vi "8-Tap 8-bit Camera with Serial Server(FPGA).vi"() -> ()   [LabVIEW 2013]
doc: "This is the FPGA VI for the 10-Tap 8-Bit Camera with DRAM example. This example demonstrates how to acquire images from a 10-tap, 8-bit, extended configuration, Camera Link camera and transfer the images to the host. This example supports area scan and line scan cameras for both continuous and finite acquisitions.\n\nThis example also demonstrates the use of DRAM as a frame buffer for very high speed acquisitions. Data packing and flow-control are also employed to maximize use of the available DRAM and FIFOs in terms of both memory space and performance.\n\nAdditionally, the example demonstrates the serial server, which allows third-party camera configuration utilities to communicate with the camera using the Camera Link serial interface while this VI is running."
uses:
  Common/CL Signal Mapping.ctl
  Common/CL Configuration.ctl
  FPGA/Sector/Accumulate/Sector Parameter Cluster.ctl
  <vilib>/Platform/TimedLoop/XDataNode/timing_clust.ctl
  <vilib>/Platform/TimedLoop/XDataNode/nitl_modes.ctl
  <vilib>/Platform/TimedLoop/XDataNode/wakeup.ctl
  <vilib>/rvi/Emulation/niFpgaSctlEmulationGetInTimedLoop.vi
  <vilib>/rvi/Emulation/niFpgaEmulationReportErrorSimple.vi
  <vilib>/rvi/eio/common/nirviEmuTemplateMethod_errors.vi
  <vilib>/rvi/Emulation/niFpgaGetClockAttributes.vi
  <vilib>/rvi/Emulation/niFpgaCriticalErrorInLSC.vi
  FPGA/Globals/Sector Parameter Global.vi
  Common/CL Data to Pixels/8 Tap 8-Bit.vi
  <vilib>/rvi/FIFO/Fifo_Resource/nirvififoEmulationWriteFpgaImpl.vi
  <vilib>/rvi/DataTransferAndStorage/Container/Common/niFpgaContainerGetUniqueNameForEmu.vi
  <vilib>/rvi/interface/RandomDataEmulation/nirviRandomDataFPGAFIFO.vi
  <vilib>/rvi/interface/RandomDataEmulation/niFpgaRandomDataHandleErrors.vi
  <vilib>/rvi/FIFO/Fifo_Resource/nirvififoEmulationGetNumberOfElementsToReadFpgaImpl.vi
  <vilib>/rvi/FIFO/Fifo_Resource/nirvififoEmulationGetNumberOfElementsToWriteFpgaImpl.vi
  <vilib>/rvi/FIFO/Fifo_Resource/nirvififoEmulationReadFpgaImpl.vi
  <vilib>/rvi/Emulation/niFpgaProcessEmulError.vi
  FPGA/Globals/Pixel Location Global.vi
  FPGA/Globals/Accumulated Sector Intensity.vi
  <vilib>/Platform/TimedLoop/XDataNode/XDataNode.xnode
  <vilib>/eio/EIONode/EIONode.xnode
  <vilib>/rvi/DataTransferAndStorage/Container/XNode/niFpgaContainer.xnode
  <vilib>/rvi/FIFO/Fifo_Resource/nirvififoEmulationWrite.vi
  <vilib>/rvi/interface/RandomDataEmulation/nirviRandomDataFpgaReadWriteTemplate.vi
  <vilib>/rvi/FIFO/Fifo_Resource/nirvififoEmulationGetNumberOfElementsToRead.vi
  <vilib>/rvi/FIFO/Fifo_Resource/nirvififoEmulationGetNumberOfElementsToWrite.vi
  <vilib>/rvi/FIFO/Fifo_Resource/nirvififoEmulationRead.vi
  <vilib>/Platform/TimedLoop/XDataNode/XDNodeRunTimeDep.lvlib
panel:
  out "Analysis Ticks":u32
  out "Right Sector Edge":u8
  out "Left Sector Edge":u8
  in  "# of Frames to Average":u8
  in  "Sector Parameters Left":T1={"Start Angle"=0.65740966796875, "End Angle"=0.99468994140625, "Inner Radius"=309, "Outter Radius"=405, "Hinge X"=464, "Hinge Y"=534, "NumWingSectors"=8}
  in  "Sector Parameters Right":T1={"Start Angle"=0.0, "End Angle"=0.4708251953125, "Inner Radius"=309, "Outter Radius"=405, "Hinge X"=685, "Hinge Y"=527, "NumWingSectors"=8}
  in  "Sector Threshold":u8
  in  "[Average BG Intensity]":u8[](array[numeric])=[0, 0, 0, 0, 0, 0, 0, 0, 0, 0, 0, 0, 0, 0, 0, 0, 0, 0, 0, 0, 0, 0, 0, 0, 0, 0, 0, 0, 0, 0, 0, 0]
  in  "X Resolution":u16=1000
  in  "Y Resolution":u16=1000
  in  "Left Start Angle Duty Cycle":fxp<+,8,0>
  in  "Left End Angle Duty Cycle":fxp<+,8,0>
  in  "Right Start Angle Duty Cycle":fxp<+,8,0>
  in  "Right End Angle Duty Cycle":fxp<+,8,0>
  out "Number of Elements to Write Host DMA":u32
  out "Number of Elements to Read Cam Data":u32
  in  "CL Config.Configuration":T2=enum."Full"
  in  "CL Config.Signal Mapping":T3
  in  "CL Config.Line Scan":bool
  in  "CL Config.DVAL Active High":bool=TRUE
  in  "CL Config.LVAL Active High":bool=TRUE
  in  "CL Config.FVAL Active High":bool=TRUE
  in  "CL Config.Spare Active High":bool=TRUE
  in  "Acq Control.Line Scan Height":u32
  in  "Acq Control.Frames To Acq":u32
  in  "Acq Control.Acquire":bool
  in  "Acq Control.Cancel Acq":bool
  in  "Acq Control.Ignore DVAL":bool
  in  "Acq Control.Initialize":bool
  out "Acq Status.Acq In Progress":bool
  out "Acq Status.Clocks Per Line":u32
  out "Acq Status.Frames Acq'd":u32
  out "Acq Status.Lines Per Frame":u32
  out "Acq Status.DMA Write Timeout":bool
  out "Acq Status.Initialized":bool
  in  "UART.Baud Rate":u8
  in  "UART.Transmit":bool
  in  "UART.Tx Data":u8[](array[numeric])=[0, 0, 0, 0, 0, 0, 0, 0, 0, 0] format="%02x"
  in  "UART.Set Baud Rate":bool
  in  "UART.Byte Mode":bool=TRUE
  out "UART.Rx Ready":bool
  out "UART.Break Indicator":bool
  out "UART.Framing Error":bool
  out "UART.Overrun Error":bool
  out "UART.Tx Ready":bool
  out "UART.Rx Data":u8 format="%02x"
  in  "UART.Receive":bool
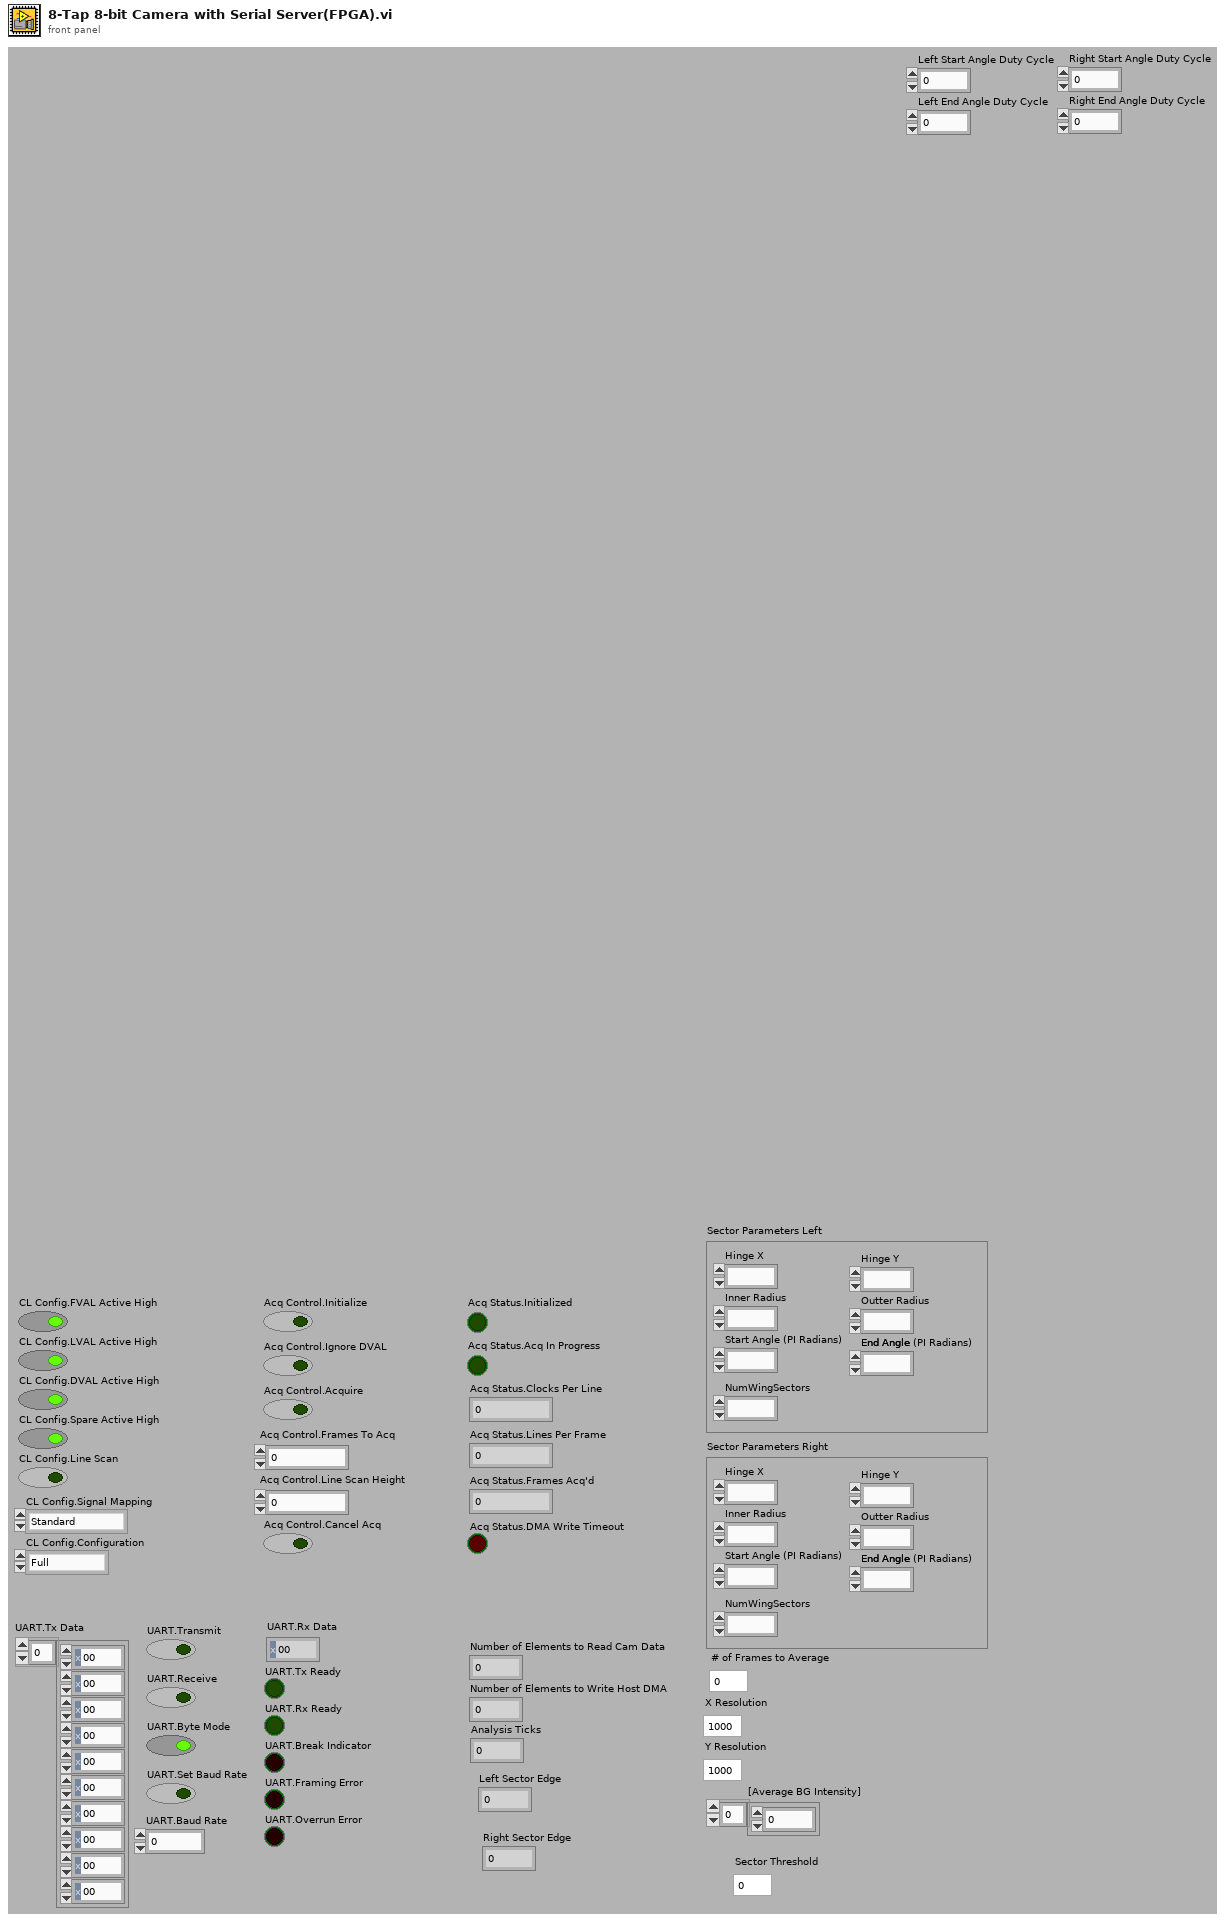
[diagram p1: front panel]
types:
  T1 = typedef "Sector Parameter Cluster.ctl" = cluster{"Start Angle":fxp<+/-,17,2>, "End Angle":fxp<+,17,3>, "Inner Radius":u16, "Outter Radius":u16, "Hinge X":u16, "Hinge Y":u16, "NumWingSectors":u8}
  T2 = typedef "CL Configuration.ctl" = enum8{"Base", "Medium", "Full"}
  T3 = typedef "CL Signal Mapping.ctl" = enum8{"Standard", "Basler 10-tap", "Vosskühler 10-tap"}
  T4 = typedef "XDNodeRunTimeDep.lvlib/timing_clust.ctl" = cluster{"Expected End [f-1]":u64, "Actual End [f-1]":u64, "Finished Late? [f-1]":bool, "Expected End [i-1]":u64, "Actual End [i-1]":u64, "Finished Late? [i-1]":bool, "Expected Start [i]":u64, "Actual Start [i]":u64, "Expected Start [f]":u64, "Actual Start [f]":u64, "Source Name":string, "Structure Name":string, "Period":i64, "Deadline":i64, "Offset":i64, "Start":i64, "Priority":i32, "Timeout":i32, "Mode":T5, "Wakeup Reason":T6, "Error":errorcluster, "Source Type":string, "Secondary Source Type":string, "Global End Time":u64, "Global Start Time":u64, "Frame Duration":u64, "Iteration Duration":u64, "Assigned CPU":i32, "I/O Scan Engine Mode":u32}
  T5 = typedef "XDNodeRunTimeDep.lvlib/nitl_modes.ctl" = enum32{"No Change", "Process missed periods, maintain original phase", "Discard missed periods, maintain original phase", "Process missed periods, ignore original phase", "Discard missed periods, ignore original phase"}
  T6 = typedef "XDNodeRunTimeDep.lvlib/wakeup.ctl" = enum32{"Normal", "Aborted", "Asynchronous wakeup", "Timing source error", "Timed loop error", "Timeout"}
  T7 = cluster{"Enables Valid":bool, "Frame Valid":bool, "Line Valid":bool, "Data Valid":bool}
  T8 = cluster{"Pixel 0":u8, "Pixel 1":u8, "Pixel 2":u8, "Pixel 3":u8, "Pixel 4":u8, "Pixel 5":u8, "Pixel 6":u8, "Pixel 7":u8}
  T9 = cluster{"Tx Data":u8[], "Transmit":bool, "Receive":bool, "Byte Mode":bool, "Set Baud Rate":bool, "Baud Rate":u8}
  T10 = cluster{"Rx Data":u8, "Turn Off Transmit":bool, "Turn Off Receive":bool, "Turn Off Set Baud Rate":bool, "Tx Ready":bool, "Rx Ready":bool, "Break Indicator":bool, "Framing Error":bool, "Overrun Error":bool}
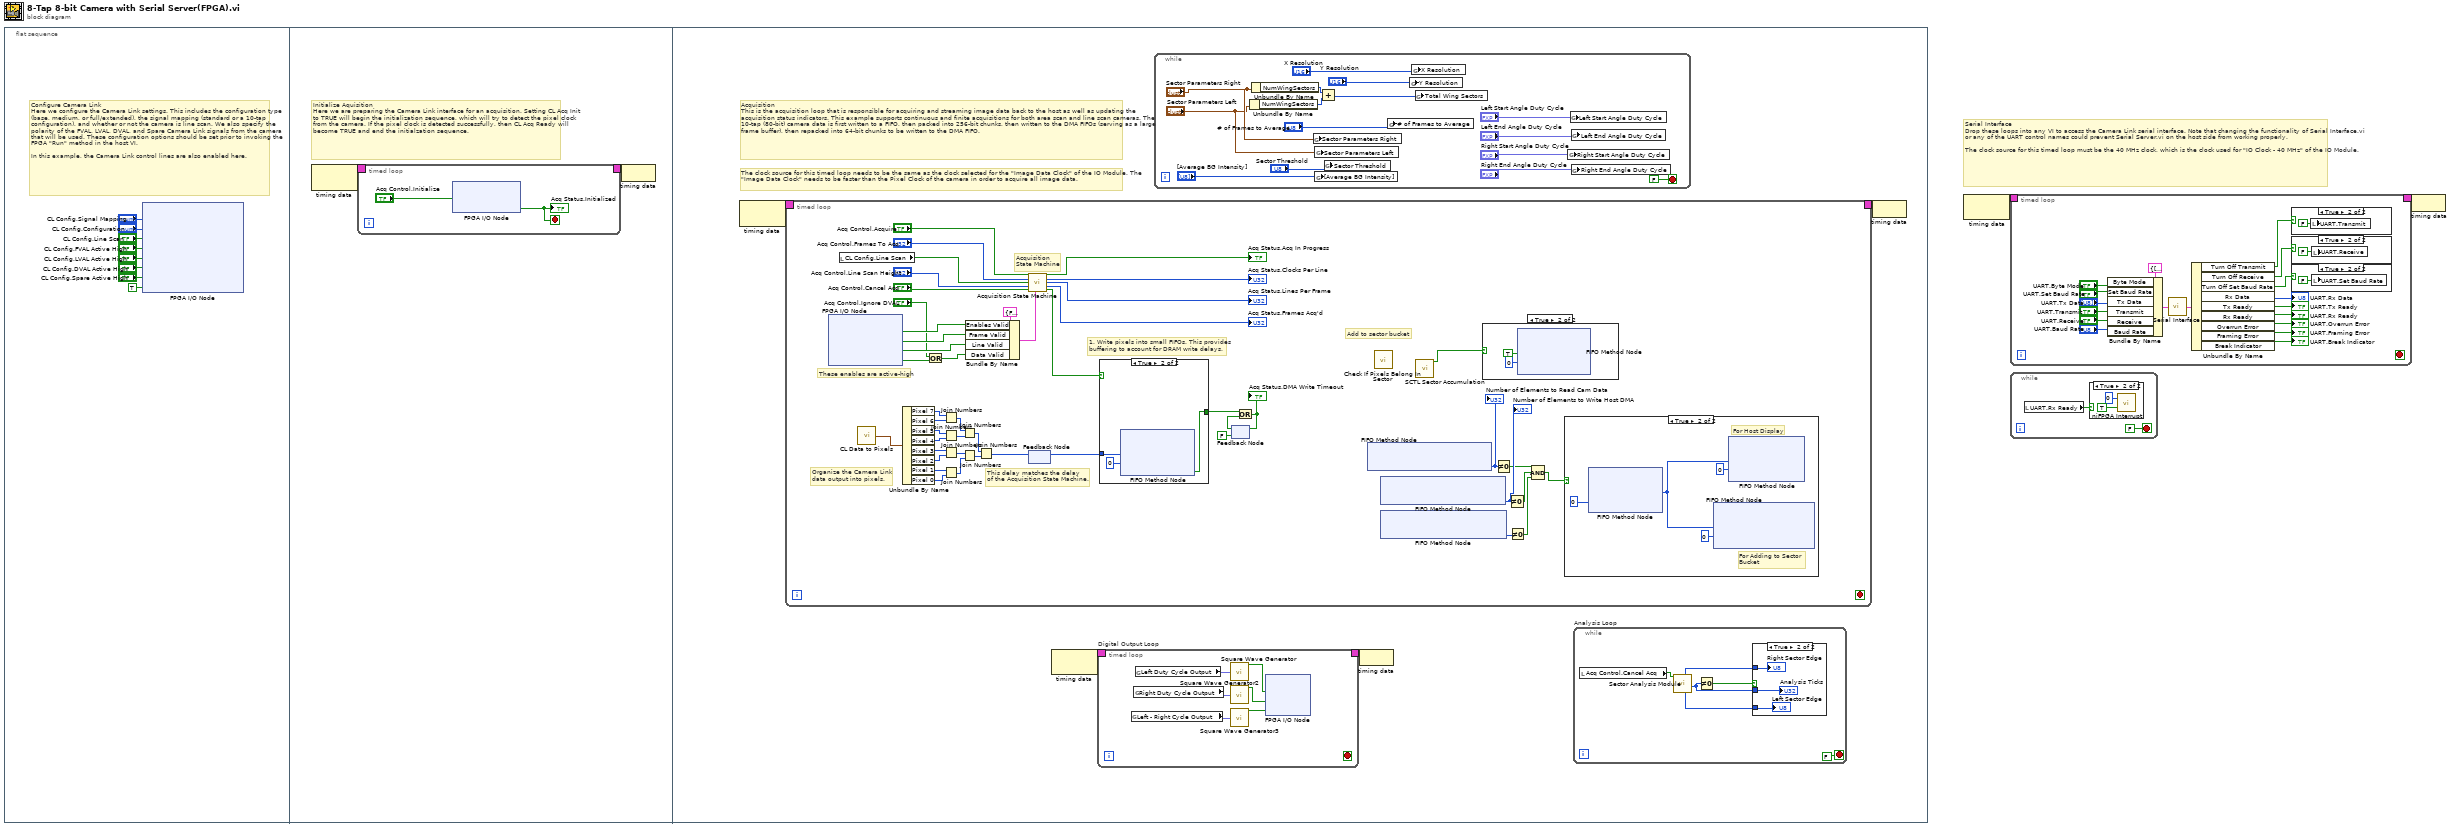
[diagram p0: block diagram]
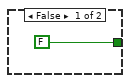
[diagram p9: hidden frame]
diagram:
  # "Serial Interface\nDrop these loops into any VI to access the Camera Link serial interface. Note that changing the functionality of Serial Interface.vi or any of the UART control names could prevent Serial Server.vi on the host side from working properly.\n\nThe clock source for this timed loop must be the 40 MHz clock, which is the clock used for \"IO Clock - 40 MHz\" of the IO Module."
  n1 = flat-sequence {
    frame #0 {
      # "Configure Camera Link\nHere we configure the Camera Link settings. This includes the configuration type (base, medium, or full/extended), the signal mapping (standard or a 10-tap configuration), and whether or not the camera is line scan. We also specify the polarity of the FVAL, LVAL, DVAL, and Spare Camera Link signals from the camera that will be used. These configuration options should be set prior to invoking the FPGA \"Run\" method in the host VI.\n\nIn this example, the Camera Link control lines are also enabled here."
      n2 = xnode "FPGA I/O Node"("CL Set Signal Mapping"="CL Config.Signal Mapping", "CL Set Configuration"="CL Config.Configuration", "CL Set Line Scan"="CL Config.Line Scan", "CL Set FVAL Active High"="CL Config.FVAL Active High", "CL Set LVAL Active High"="CL Config.LVAL Active High", "CL Set DVAL Active High"="CL Config.DVAL Active High", "CL Set Spare Active High"="CL Config.Spare Active High", "CL Control Enable"=TRUE ("IO Module\\CL Control Enable")) -> ()  [unwired: 8 in, 8 out]
    }
    frame #1 {
      # "Initialize Aquisition\nHere we are preparing the Camera Link interface for an acquisition. Setting CL Acq Init to TRUE will begin the initialization sequence, which will try to detect the pixel clock from the camera. If the pixel clock is detected successfully, then CL Acq Ready will become TRUE and end the initialzation sequence."
      n3 = node-c288() -> (w12:T4)  [unwired: 1 out]
      n4 = timed-loop {
        timing: w12 -> [_]
        timing-out: [_] -> w11
        stop <- w13 stop-if-true
        n5 = xnode "FPGA I/O Node"("CL Acq Init"="Acq Control.Initialize") -> ("CL Acq Ready"=w13:bool)  [unwired: 2 in, 2 out]
        "Acq Status.Initialized" <- w13
      }
      n6 = node-c288(w11) -> ()
    }
    frame #2 {
      # "The clock source for this timed loop needs to be the same as the clock selected for the \"Image Data Clock\" of the IO Module. The \"Image Data Clock\" needs to be faster than the Pixel Clock of the camera in order to acquire all image data."
      # "Acquisition\nThis is the acquisition loop that is responsible for acquiring and streaming image data back to the host as well as updating the acquisition status indicators. This example supports continuous and finite acquisitions for both area scan and line scan cameras. The 10-tap (80-bit) camera data is first written to a FIFO, then packed into 256-bit chunks, then written to the DMA FIFOs (serving as a large frame buffer), then repacked into 64-bit chunks to be written to the DMA FIFO."
      n7 = node-c288() -> (w22:T4)  [unwired: 1 in]
      n8 = timed-loop {
        timing: w22 -> [_]
        timing-out: [_] -> w21
        stop <- _ stop-if-true
        # "Add to sector bucket"
        # "1. Write pixels into small FIFOs. This provides\nbuffering to account for DRAM write delays."
        # "Organize the Camera Link\ndata output into pixels."
        # "These enables are active-high"
        # "This delay matches the delay\nof the Acquisition State Machine."
        # "Acquisition\nState Machine"
        n9 = xnode "FPGA I/O Node"() -> ("CL Output Valid"=w89:bool, "CL Frame Valid"=w88:bool, "CL Line Valid"=w87:bool, "CL Data Valid"=w84:bool)  [unwired: 4 in, 4 out]
        n10 = local read "CL Config.Line Scan"() -> (w81:bool)
        n11 = call-poly "CL Data to Pixels.vi"() -> ("Pixels"=w103:T8)  [unwired: 1 in]
        n12 = Unbundle By Name(w103) -> ("Pixel 7"=w79:u8, "Pixel 6"=w78:u8, "Pixel 5"=w77:u8, "Pixel 4"=w76:u8, "Pixel 3"=w75:u8, "Pixel 2"=w74:u8, "Pixel 1"=w73:u8, "Pixel 0"=w72:u8)
        n13 = Or(x="Acq Control.Ignore DVAL", y=w84) -> (x .or. y?=w83:bool)
        n14 = Join Numbers(hi=w79, lo=w78) -> ((hi.lo)=w70:u16)
        n15 = Join Numbers(hi=w77, lo=w76) -> ((hi.lo)=w69:u16)
        n16 = Join Numbers(hi=w75, lo=w74) -> ((hi.lo)=w68:u16)
        n17 = Join Numbers(hi=w73, lo=w72) -> ((hi.lo)=w71:u16)
        n18 = Join Numbers(hi=w70, lo=w69) -> ((hi.lo)=w67:u32)
        n19 = Join Numbers(hi=w68, lo=w71) -> ((hi.lo)=w66:u32)
        n20 = Bundle By Name(cluster=T7 {"Enables Valid"=FALSE, "Frame Valid"=FALSE, "Line Valid"=FALSE, "Data Valid"=FALSE} ("Enables"), "Enables Valid"=w89, "Frame Valid"=w88, "Line Valid"=w87, "Data Valid"=w83) -> (w86:T7)
        n21 = Join Numbers(hi=w67, lo=w66) -> ((hi.lo)=w65:u64)
        n22 = call "Acquisition State Machine.vi"("Acquire"="Acq Control.Acquire", "Frames to Acquire"="Acq Control.Frames To Acq", "Line Scan"=w81, "Line Scan Height"="Acq Control.Line Scan Height", "Cancel Acq"="Acq Control.Cancel Acq", "Enables"=w86) -> ("Acq In Progress"=→"Acq Status.Acq In Progress":bool, "Num Clocks Per Line"=→"Acq Status.Clocks Per Line":u32, "Num Lines Per Frame"=→"Acq Status.Lines Per Frame":u32, "Num Frames Acq'd"=→"Acq Status.Frames Acq'd":u32, "Capture Cycle"=w101:bool)  [unwired: 4 in, 1 out]
        n23 = feedback-in #1(w65) -> ()
        n24 = feedback #1() -> (w102:u64)  [unwired: 1 in]
        n25 = case shown="True" w101 {
          tunnel: [FALSE ("Timed Out?") w112] -> w99
          tunnel: w102 -> [_ w113]
          frame False {
          }
          frame True {
            n26 = xnode ("FIFO Method Node")("Element"=w113, "Timeout"=0) -> ("Timed Out?"=w112:bool)  [unwired: 1 in, 1 out]
          }
        }
        n27 = feedback #2(FALSE) -> (w98:bool)
        n28 = Or(x=w99, y=w98) -> (x .or. y?=w97:bool)
        "Acq Status.DMA Write Timeout" <- w97
        n29 = feedback-in #2(w97) -> ()
        n30 = xnode ("FIFO Method Node")() -> ("Number of Elements to Read"=w63:u32)  [unwired: 1 in, 1 out]
        "Number of Elements to Read Cam Data" <- w63
        n31 = call "Check If Pixels Belong In Sector.vi"() -> ()  [unwired: 11 in, 1 out]
        n32 = xnode ("FIFO Method Node")() -> ("Number of Elements to Write"=w61:u32)  [unwired: 1 in, 1 out]
        "Number of Elements to Write Host DMA" <- w61
        n33 = xnode ("FIFO Method Node")() -> ("Number of Elements to Write"=w60:u32)  [unwired: 1 in, 1 out]
        n34 = call "SCTL Sector Accumulation.vi"() -> ("New Data?"=w64:bool)  [unwired: 10 in, 1 out]
        n35 = case shown="True" w64 {
          frame False {
          }
          frame True {
            n36 = xnode ("FIFO Method Node")("Element"=TRUE, "Timeout"=0) -> ()  [unwired: 1 in, 2 out]
          }
        }
        n37 = Not Equal To 0?(x=w63) -> (x != 0?=w58:bool)
        n38 = Not Equal To 0?(x=w61) -> (x != 0?=w62:bool)
        n39 = Not Equal To 0?(x=w60) -> (x != 0?=w59:bool)
        n40 = Compound Arithmetic op=AND(w58, w62, w59) -> (w57:bool)
        n41 = case shown="True" w57 {
          frame False {
          }
          frame True {
            # "For Adding to Sector \nBucket"
            # "For Host Display"
            n42 = xnode ("FIFO Method Node")("Timeout"=0) -> ("Element"=w104:u64)  [unwired: 1 in, 2 out]
            n43 = xnode ("FIFO Method Node")("Element"=w104, "Timeout"=0) -> ()  [unwired: 1 in, 2 out]
            n44 = xnode ("FIFO Method Node")("Element"=w104, "Timeout"=0) -> ()  [unwired: 1 in, 2 out]
          }
        }
      }
      n45 = node-c288() -> (w20:T4)  [unwired: 1 in]
      n46 = timed-loop "Digital Output Loop" {
        timing: w20 -> [_]
        timing-out: [_] -> w19
        stop <- _ stop-if-true
        n47 = global read "Sector Parameter Global.vi" "Left - Right Cycle Output"() -> (w50:fxp<+,8,0>)
        n48 = global read "Sector Parameter Global.vi" "Right Duty Cycle Output"() -> (w51:fxp<+,8,0>)
        n49 = global read "Sector Parameter Global.vi" "Left Duty Cycle Output"() -> (w52:fxp<+,8,0>)
        n50 = call "Square Wave Generator"("duty cycle (periods)"=w52) -> ("square wave out"=w49:bool)  [unwired: 14 in]
        n51 = call "Square Wave Generator2"("duty cycle (periods)"=w51) -> ("square wave out"=w48:bool)  [unwired: 14 in]
        n52 = call "Square Wave Generator3"("duty cycle (periods)"=w50) -> ("square wave out"=w47:bool)  [unwired: 14 in]
        n53 = xnode "FPGA I/O Node"("TTL 0"=w49, "TTL 1"=w48, "TTL 2"=w47) -> ()  [unwired: 3 in, 3 out]
      }
      n54 = while {
        stop <- FALSE stop-if-true
        n55 = Unbundle By Name("Sector Parameters Left") -> ("NumWingSectors"=w44:u8)
        n56 = Unbundle By Name("Sector Parameters Right") -> ("NumWingSectors"=w45:u8)
        n57 = global write "Sector Parameter Global.vi" "Sector Parameters Right"("Sector Parameters Right") -> ()
        n58 = global write "Sector Parameter Global.vi" "Sector Parameters Left"("Sector Parameters Left") -> ()
        n59 = global write "Sector Parameter Global.vi" "[Average BG Intensity]"("[Average BG Intensity]") -> ()
        n60 = Add(x=w45, y=w44) -> (x+y=w43:u8)
        n61 = global write "Sector Parameter Global.vi" "Sector Threshold"("Sector Threshold") -> ()
        n62 = global write "Pixel Location Global.vi" "# of Frames to Average"("# of Frames to Average") -> ()
        n63 = global write "Pixel Location Global.vi" "Y Resolution"("Y Resolution") -> ()
        n64 = global write "Pixel Location Global.vi" "X Resolution"("X Resolution") -> ()
        n65 = global write "Accumulated Sector Intensity.vi" "Total Wing Sectors"(w43) -> ()
        n66 = global write "Sector Parameter Global.vi" "Right Start Angle Duty Cycle"("Right Start Angle Duty Cycle") -> ()
        n67 = global write "Sector Parameter Global.vi" "Left Start Angle Duty Cycle"("Left Start Angle Duty Cycle") -> ()
        n68 = global write "Sector Parameter Global.vi" "Left End Angle Duty Cycle"("Left End Angle Duty Cycle") -> ()
        n69 = global write "Sector Parameter Global.vi" "Right End Angle Duty Cycle"("Right End Angle Duty Cycle") -> ()
      }
      n70 = node-c288(w19) -> ()
      n71 = while "Analysis Loop" {
        stop <- FALSE stop-if-true
        n72 = local read "Acq Control.Cancel Acq"() -> (w27:bool)
        n73 = call "Sector Analysis Module.vi"("Canceled?"=w27) -> ("Analysis Ticks"=w26:u32, "Left Sector Edge"=w23:u8, "Right Sector Edge"=w24:u8)  [unwired: 6 in, 2 out]
        n74 = Not Equal To 0?(x=w26) -> (x != 0?=w25:bool)
        n75 = case shown="True" w25 {
          tunnel: w26 -> [_ w31]
          tunnel: w24 -> [_ w30]
          tunnel: w23 -> [_ w29]
          frame False {
          }
          frame True {
            "Analysis Ticks" <- w31
            "Right Sector Edge" <- w30
            "Left Sector Edge" <- w29
          }
        }
      }
      n76 = node-c288(w21) -> ()
    }
  }
  n77 = node-c288() -> (w2:T4)  [unwired: 1 out]
  n78 = timed-loop {
    timing: w2 -> [_]
    timing-out: [_] -> w1
    stop <- _ stop-if-true
    n79 = Bundle By Name(cluster=T9 {"Tx Data"=[0, 0, 0, 0, 0, 0, 0, 0, 0, 0], "Transmit"=FALSE, "Receive"=FALSE, "Byte Mode"=TRUE, "Set Baud Rate"=FALSE, "Baud Rate"=0} ("UART Inputs"), "Byte Mode"="UART.Byte Mode", "Set Baud Rate"="UART.Set Baud Rate", "Tx Data"="UART.Tx Data", "Transmit"="UART.Transmit", "Receive"="UART.Receive", "Baud Rate"="UART.Baud Rate") -> (w118:T9)
    n80 = call "Serial Interface.vi"("UART Inputs"=w118) -> ("UART Outputs"=w130:T10)
    n81 = Unbundle By Name(w130) -> ("Turn Off Transmit"=w123:bool, "Turn Off Receive"=w124:bool, "Turn Off Set Baud Rate"=w120:bool, "Rx Data"=→"UART.Rx Data":u8, "Tx Ready"=→"UART.Tx Ready":bool, "Rx Ready"=→"UART.Rx Ready":bool, "Overrun Error"=→"UART.Overrun Error":bool, "Framing Error"=→"UART.Framing Error":bool, "Break Indicator"=→"UART.Break Indicator":bool)
    n82 = case shown="True" w123 {
      frame False {
      }
      frame True {
        n83 = local write "UART.Transmit"(FALSE ("UART.Transmit")) -> ()
      }
    }
    n84 = case shown="True" w124 {
      frame False {
      }
      frame True {
        n85 = local write "UART.Receive"(FALSE ("UART.Receive")) -> ()
      }
    }
    n86 = case shown="True" w120 {
      frame False {
      }
      frame True {
        n87 = local write "UART.Set Baud Rate"(FALSE ("UART.Receive")) -> ()
      }
    }
  }
  n88 = while {
    stop <- FALSE stop-if-true
    n89 = local read "UART.Rx Ready"() -> (w142:bool)
    n90 = case shown="True" w142 {
      frame False {
      }
      frame True {
        n91 = call <vilib>:"niFPGA Interrupt.vi"("Wait Until Cleared (F)"=TRUE ("Wait Until Cleared"), "IRQ Number (0)"=u8 0 ("IRQ Number")) -> ()  [unwired: 1 in]
      }
    }
  }
  n92 = node-c288(w1) -> ()
